vi "TSCAN_Disconnect.vi"(8 "错误输入（无错误）":errorcluster, 11 "路径输入":path) -> (0 "错误输出":errorcluster, 3 "路径输出":path)   [LabVIEW 2019]
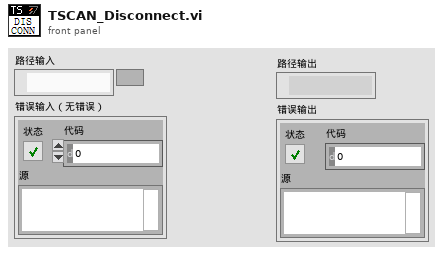
[diagram p1: front panel]
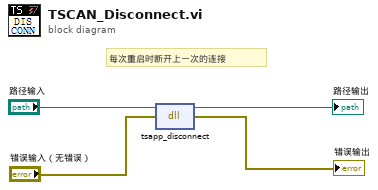
[diagram p0: block diagram]
diagram:
  # "每次重启时断开上一次的连接"
  n1 = dll-call lib="PTH2Zabs CUsers\nAdministratorDesktopLB2018TS_CAN通讯 文件夹PathTSMaster.dll" fn="tsapp_disconnect"(path in="路径输入", error in="错误输入（无错误）") -> (path out=→"路径输出":path, error out=→"错误输出":errorcluster)  [unwired: 2 in]
